vi "AlliGator Compute Natural Frequency.vi"(8 "Error In":errorcluster) -> (0 "Error Out":errorcluster, 3 "Natural Frequency":dbl[unit] caption="Laser Period" min=0.0 format="%#.3g")   [LabVIEW 2021, in "AlliGator Settings.lvlib"]
doc: "Computes the \"natural\" phasor frequency as a functions of various settings parameters."
uses:
  AlliGator Settings.lvlib
  AlliGator Settings List.ctl
  AlliGator Background Subtraction Parameters.ctl
  Graphs/XY Graph/XY Graph Plot Shift Parameters.ctl
  Graphs/XY Graph/XY Graph Plot Shift Method.ctl
  Variant/Variant to Data/Variant to U32.vi
  Variant/Variant to Data/Variant to Boolean.vi
  Variant/Variant to Data/Variant to Data.lvlib
  Graphs/XY Graph/XY Graph Add-Ons.lvlib
panel:
  # "see the AlliGator License on the block diagram (Ctrl+E or Window:Show Block Diagram)"
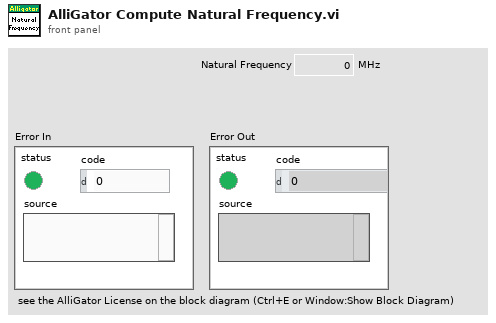
[diagram p1: front panel]
types:
  T1 = typedef "AlliGator Settings.lvlib/AlliGator Settings List.ctl" = enum16{"GUI:Visible Settings Tab", "GUI:Last Run Version", "Source Image:Use Image Histogram for Contrast", "Source Image:Low Count Pixels Rejection Options", "Source Image:High Count Pixels Rejection Options", "Source Image:Use Image Brightness", "Source Image:Blend Overlay with Image Background", "Source Image:Use Fixed ROI Diameter", "Source Image:ROI Diameter", "Source Image:ROI Center Color", "Source Image:Peak Threshold", "Source Image:Intensity Threshold", "Source Image:Image Binning Options", "Source Image:Image Smoothing Options", "Source Image:Image Histogram Active", "Source Image:Invert Binary Mask", "Source Image:Hot Pixel Removal", "Source Image:Overlay Analyzed ROI Center", "Source Image:Auto-Adjust Contrast", "Source Image:Histogram Lower Percentile", "Source Image:Histogram Upper Percentile", "Source Image:Save Source Image", "Source Image:Scale Bar Options", "Source Image:Image Resolution (Pixel Size)", "Source Image:Flatfield Correction", "Source Image:Show Dead Left Columns Correction", "Source Image:Dead Left Columns Correction", "Source Image:Image Pre-Processing Operations Order", "Source Image:Overlay ROI Median", "Source Image:Median Overlay Color", "Data Information:Gate Width", "Data Information:Nanotime Gate Separation", "Data Information:Macrotime Gate Separation", "Data Information:Gate Step", "Data Information:# Gates", "Data Information:Gate Image Exposure", "Data Information:Gate Image Integration", "Data Information:Gates to Skip", "Data Information:Gates to Keep", "Data Information:Define Gates to", "Data Information:Channel Name", "Data Information:Available Channel Names", "Data Information:Channel Arithmetic", "Data Information:Background File Subtraction", "Data Information:Background File", "Data Information:Background Scaling Factor", "Data Information:Background Pile-up Correction", "Data Information:Background Pixel Well Capacity", "Data Information:Laser Period", "Data Information:SYNC Period", "Data Information:Pile-up Correction", "Data Information:Pixel Well Capacity", "Data Information:Dataset Scaling Factor", "Fluorescence Decay_Decay Pre-Processing:Reverse Gates", "Fluorescence Decay_Decay Pre-Processing:Verbose Decay Pre-Processing", "Fluorescence Decay_Decay Pre-Processing:Use Decay Pre-Processing", "Fluorescence Decay_Decay Pre-Processing:Background Subtraction", "Fluorescence Decay_Decay Pre-Processing:Background Definition Range", "Fluorescence Decay_Decay Pre-Processing:Baseline Subtraction Method", "Fluorescence Decay_Decay Pre-Processing:Decay Pre-Processing Operations Order", "Fluorescence Decay_Decay Pre-Processing:Smoothing Parameter", "Fluorescence Decay_Decay Pre-Processing:Shift Decay", "Fluorescence Decay_Decay Pre-Processing:Decay Shift Parameters", "Fluorescence Decay_Decay Pre-Processing:Fold Decay", "Fluorescence Decay_Decay Pre-Processing:# Folds", "Fluorescence Decay_Decay Pre-Processing:1-Normalize Decay", "Fluorescence Decay_Decay Pre-Processing:[0-1]-Normalize Decay", "Fluorescence Decay_Decay Pre-Processing:Smoothen Decay", "Fluorescence Decay_Decay Pre-Processing:Extrapolate Decay", "Fluorescence Decay_Decay Pre-Processing:Use Periodicity", "Fluorescence Decay_Decay Pre-Processing:Use Cursors", "Fluorescence Decay_Decay Pre-Processing:Tail Fraction", "Fluorescence Decay_Decay Pre-Processing:Head Fraction", "Fluorescence Decay_Decay Pre-Processing:Additional Points", "Fluorescence Decay_Decay Pre-Processing:Straighten Decay", "Fluorescence Decay_Decay Pre-Processing:Constant Background", "Fluorescence Decay_Decay Pre-Processing:Pixel-Normalize Decay", "Fluorescence Decay_Advanced Analysis:Extract IRF instead of Decay", "Fluorescence Decay_Advanced Analysis:IRF Extraction Options", "Fluorescence Decay_Advanced Analysis:IRF Optimization Options", "Fluorescence Decay_Advanced Analysis:Square Pulse Options", "Fluorescence Decay_Advanced Analysis:IRF Order", "Fluorescence Decay_Advanced Analysis:IRF Time Constants", "Fluorescence Decay_Advanced Analysis:Wavelet Analysis Options", "Fluorescence Decay_Advanced Analysis:Average Lifetime Options", "Fluorescence Decay_Fit Options:Fit Options", "Fluorescence Decay_Fit Options:Use Legacy Fitting Approach", "Fluorescence Decay_Fit Options:Use Data Information Laser Period", "Fluorescence Decay_Fit Parameters:Displayed Fit Parameters", "Fluorescence Decay_Fit Parameters:Fit Parameter Constraints", "Fluorescence Decay_Fit Parameters:Export Tabulated Results", "Fluorescence Decay_Fit Parameters:MLE Baseline Offset Type", "Fluorescence Decay_Fit Parameters:MLE Baseline Offset", "Fluorescence Decay_Fit Parameters:Guess Parameter Names", "Fluorescence Decay_Fit Parameters:Guess Parameter Values", "Fluorescence Decay_Fit Parameters:Guess Parameters Options", "Fluorescence Decay_Styles:Show Last Decay Only", "Fluorescence Decay_Styles:Decay Graph Color Array", "Fluorescence Decay:Decay Graph Active", "Fluorescence Decay Statistics:Min Peak Value", "Fluorescence Decay Statistics:Reject Low Decay Peak Pixels", "Fluorescence Decay Statistics:Reject High Decay Peak Pixels", "Fluorescence Decay Statistics:Max Peak Value", "Time Traces:Use File Timestamp", "Time Traces:Time Step", "Time Traces:Use Intensity Correction File", "Time Traces:Intensity Correction File", "Phasor Plot:Phasor Plot Smoothing Options", "Phasor Plot:Phasor Plot Size", "Phasor Plot:Phasor Plot Graphics Options", "Phasor Plot:Cumulative Phasor Plot", "Phasor Plot:Use Phasor Brightness", "Phasor Plot:Blend Overlay with Phasor Background", "Phasor Plot:Save Phasor Plot", "Phasor Plot:Show References", "Phasor Plot:Phasor Ratio Decay Range", "Phasor Plot:Exponential Fading", "Phasor Plot:Phasor Ratio Reference Colors", "Phasor Plot:Reference Radius", "Phasor Plot:Show Color Map Vertices", "Phasor Plot:Phasor Plot Active", "Phasor Plot:Phasor Ratio Color Map Type", "Phasor Plot:Phasor Ratio Color Map", "Phasor Plot:Phasor Ratio Display Range", "Phasor Plot:Selected Image ROI(s)", "Phasor Plot:All Image ROIs", "Phasor Plot:Selected Phasor Plot ROI(s)", "Phasor Plot:All Phasor Plot ROIs", "Phasor Plot:Phasor Ratio Color-Coded Quantity", "Phasor Plot:Store Phasor Harmonics", "Phasor Plot:Draw Reference Segment", "Phasor Plot:User-Defined Quantity", "Phasor Graph:Phasor Frequency", "Phasor Graph:Phasor Ratio Type", "Phasor Graph:Pixel-level Phasor Computation", "Phasor Graph:Save Phasor Graph", "Phasor Graph:Phasor Graph Active", "Phasor Graph:Phasor SDV Options", "Phasor Calibration:Use Backup Calibration if needed", "Phasor Graph:Define Shortest Lifetime as", "Phasor Calibration:Backup Calibration Type", "Phasor Calibration:Calibration Type", "Phasor Calibration:Calibration Lifetime", "Phasor Calibration:Calibration Map Algorithm", "Single-Exponential Phasor Locus (SEPL):Gate Parameters", "Single-Exponential Phasor Locus (SEPL):User-defined Gate", "Single-Exponential Phasor Locus (SEPL):User-defined IRF", "Single-Exponential Phasor Locus (SEPL):Phasor Parameters", "Single-Exponential Phasor Locus (SEPL):Decay & IRF Parameters", "Single-Exponential Phasor Locus (SEPL):Display Parameters", "Lifetime Analysis:Decay Analysis Parameters", "Lifetime Analysis:Lifetime Map Active", "Plugins:Python Settings", "Miscellaneous:Verbose Mode", "Miscellaneous:Beep after Script", "Miscellaneous:Saved Image File Format", "Miscellaneous:Exported Gate Image Settings", "Miscellaneous:Include Loading in Timing", "Miscellaneous:Verbose Settings Mode", "Miscellaneous:Histogram Options", "Miscellaneous:Beep on Error", "Miscellaneous:# Logical Processors Used", "Miscellaneous:ROI Description Max Characters", "Miscellaneous:Verbose Error Mode", "Miscellaneous:Transparent Mask Color"}
  T2 = typedef "XY Graph Add-Ons.lvlib/XY Graph Plot Shift Parameters.ctl" = cluster{"Type":T3, "Shift":dbl[unit], "Threshold":dbl, "Rotate":bool}
  T3 = typedef "XY Graph Add-Ons.lvlib/XY Graph Plot Shift Method.ctl" = enum16{"Default", "CFD", "Threshold", "Cross-Correlation"}
  T4 = typedef "AlliGator Settings.lvlib/AlliGator Background Subtraction Parameters.ctl" = cluster{"Start":u32, "End":u32}
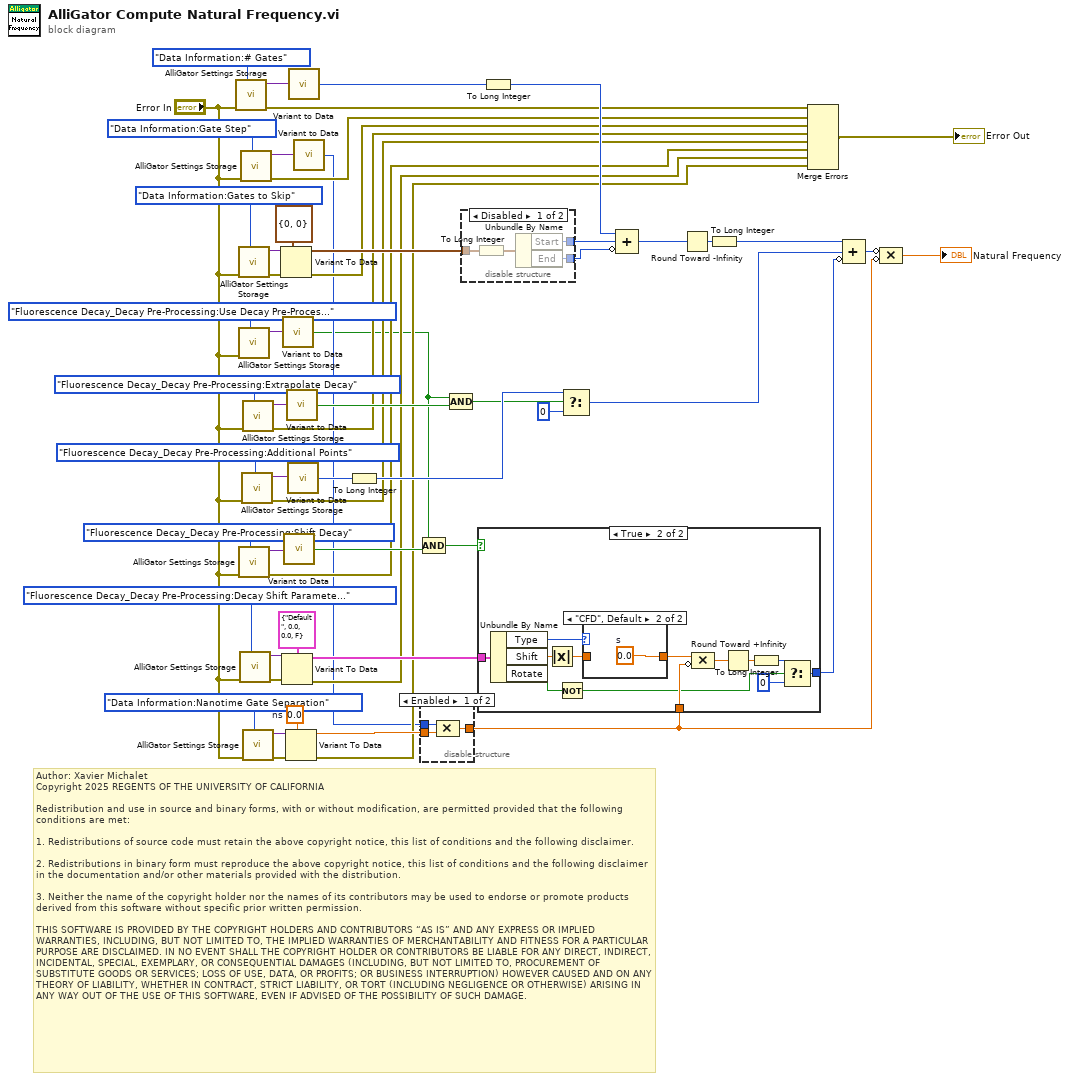
[diagram p0: block diagram]
diagram:
  w35 = dbl[unit] 0.0  # ns
  # "Author: Xavier Michalet\nCopyright 2025 REGENTS OF THE UNIVERSITY OF CALIFORNIA\n\nRedistribution and use in source and binary forms, with or without modification, are permitted provided that the following conditions are met:\n\n1. Redistributions of source code must retain the above copyright notice, this list of conditions and the following disclaimer.\n\n2. Redistributions in binary form must reproduce the above copyright notice, this list of conditions and the following disclaimer in the documentation and/or other materials provided with the distribution.\n\n3. Neither the name of the copyright holder nor the names of its contributors may be used to endorse or promote products derived from this software without specific prior written permission.\n\nTHIS SOFTWARE IS PROVIDED BY THE COPYRIGHT HOLDERS AND CONTRIBUTORS “AS IS” AND ANY EXPRESS OR IMPLIED WARRANTIES, INCLUDING, BUT NOT LIMITED TO, THE IMPLIED WARRANTIES OF MERCHANTABILITY AND FITNESS FOR A PARTICULAR PURPOSE ARE DISCLAIMED. IN NO EVENT SHALL THE COPYRIGHT HOLDER OR CONTRIBUTORS BE LIABLE FOR ANY DIRECT, INDIRECT, INCIDENTAL, SPECIAL, EXEMPLARY, OR CONSEQUENTIAL DAMAGES (INCLUDING, BUT NOT LIMITED TO, PROCUREMENT OF SUBSTITUTE GOODS OR SERVICES; LOSS OF USE, DATA, OR PROFITS; OR BUSINESS INTERRUPTION) HOWEVER CAUSED AND ON ANY THEORY OF LIABILITY, WHETHER IN CONTRACT, STRICT LIABILITY, OR TORT (INCLUDING NEGLIGENCE OR OTHERWISE) ARISING IN ANY WAY OUT OF THE USE OF THIS SOFTWARE, EVEN IF ADVISED OF THE POSSIBILITY OF SUCH DAMAGE."
  n1 = call "AlliGator Settings Storage.vi"("AlliGator Settings List"=AlliGator_Settings_List."Data Information:# Gates", "Error In"="Error In") -> ("Error Out"=w18:errorcluster, "Variant Data out"=w52:variant)  [unwired: 8 in]
  n2 = call "AlliGator Settings Storage.vi"("AlliGator Settings List"=AlliGator_Settings_List."Data Information:Gates to Skip", "Error In"="Error In") -> ("Error Out"=w50:errorcluster, "Variant Data out"=w51:variant)  [unwired: 8 in]
  n3 = call "AlliGator Settings Storage.vi"("AlliGator Settings List"=AlliGator_Settings_List."Fluorescence Decay_Decay Pre-Processing:Use Decay Pre-Processing", "Error In"="Error In") -> ("Variant Data out"=w6:variant)  [unwired: 8 in, 1 out]
  n4 = call "AlliGator Settings Storage.vi"("AlliGator Settings List"=AlliGator_Settings_List."Fluorescence Decay_Decay Pre-Processing:Shift Decay", "Error In"="Error In") -> ("Error Out"=w13:errorcluster, "Variant Data out"=w48:variant)  [unwired: 8 in]
  n5 = call "AlliGator Settings Storage.vi"("AlliGator Settings List"=AlliGator_Settings_List."Fluorescence Decay_Decay Pre-Processing:Decay Shift Parameters", "Error In"="Error In") -> ("Error Out"=w46:errorcluster, "Variant Data out"=w47:variant)  [unwired: 8 in]
  n6 = call "AlliGator Settings Storage.vi"("AlliGator Settings List"=AlliGator_Settings_List."Data Information:Gate Step", "Error In"="Error In") -> ("Error Out"=w17:errorcluster, "Variant Data out"=w40:variant)  [unwired: 8 in]
  n7 = call "AlliGator Settings Storage.vi"("AlliGator Settings List"=AlliGator_Settings_List."Fluorescence Decay_Decay Pre-Processing:Additional Points", "Error In"="Error In") -> ("Error Out"=w14:errorcluster, "Variant Data out"=w43:variant)  [unwired: 8 in]
  n8 = call "AlliGator Settings Storage.vi"("AlliGator Settings List"=AlliGator_Settings_List."Fluorescence Decay_Decay Pre-Processing:Extrapolate Decay", "Error In"="Error In") -> ("Error Out"=w15:errorcluster, "Variant Data out"=w44:variant)  [unwired: 8 in]
  n9 = call "AlliGator Settings Storage.vi"("AlliGator Settings List"=AlliGator_Settings_List."Data Information:Nanotime Gate Separation", "Error In"="Error In") -> ("Error Out"=w37:errorcluster, "Variant Data out"=w36:variant)  [unwired: 8 in]
  n10 = Variant To Data(error in=w50, type=T4 {"Start"=0, "End"=0} ("Gates to Skip"), Variant=w51) -> (data=w42:T4, error out=w16:errorcluster)
  n11 = Variant To Data(error in=w46, type=T2 {"Type"=enum."Default", "Shift"=0.0, "Threshold"=0.0, "Rotate"=FALSE} ("IRF Analysis Parameters"), Variant=w47) -> (data=w41:T2, error out=w12:errorcluster)
  n12 = call-poly "Variant to Data.vi"("Variant"=w6) -> ("Value"=w1:bool)  [unwired: 8 in]
  n13 = call-poly "Variant to Data.vi"("Variant"=w48) -> ("Value"=w30:bool)  [unwired: 8 in]
  n14 = Variant To Data(error in=w37, type=w35, Variant=w36) -> (data=w20:dbl[unit], error out=w11:errorcluster)
  n15 = call-poly "Variant to Data.vi"("Variant"=w44) -> ("Value"=w29:bool)  [unwired: 8 in]
  n16 = call-poly "Variant to Data.vi"("Variant"=w43) -> ("Value"=w28:u32)  [unwired: 8 in]
  n17 = call-poly "Variant to Data.vi"("Variant"=w52) -> ("Value"=w34:u32)  [unwired: 8 in]
  n18 = call-poly "Variant to Data.vi"("Variant"=w40) -> ("Value"=w7:u32)  [unwired: 8 in]
  n19 = To Long Integer(number=w28) -> (32bit integer=w27:i32)
  n20 = disable-structure shown="Enabled" {
    disable-tunnel: w20 -> [w61 w62]
    disable-tunnel: [w60 w62] -> w9
    disable-tunnel: w7 -> [w59 _]
    frame Enabled {
      n21 = Compound Arithmetic op=MULTIPLY(w59, w61) -> (w60:dbl[unit])
    }
    frame Disabled {
    }
  }
  n22 = Compound Arithmetic op=AND(w1, w30) -> (w3:bool)
  n23 = Compound Arithmetic op=AND(w1, w29) -> (w2:bool)
  n24 = disable-structure shown="Disabled" {
    disable-tunnel: w42 -> [w66 _]
    disable-tunnel: [w65 _] -> w33
    disable-tunnel: [w63 _] -> w31
    frame Disabled {
      n25 = To Long Integer(number=w66) -> (32bit integer=w64:cluster{"Start":i32, "End":i32})
      n26 = Unbundle By Name(w64) -> ("Start"=w65:i32, "End"=w63:i32)
    }
    frame Enabled {
    }
  }
  n27 = case shown="True" w3 {
    tunnel: w41 -> [_ w79]
    tunnel: w9 -> [_ w73]
    tunnel: [_ w68] -> w22
    frame False {
    }
    frame True {
      n28 = Unbundle By Name(w79) -> ("Type"=w78:T3, "Shift"=w77:dbl[unit], "Rotate"=w75:bool)
      n29 = Absolute Value(x=w77) -> (abs(x)=w76:dbl[unit])
      n30 = Not(x=w75) -> (.not. x?=w67:bool)
      n31 = case shown="\"CFD\", Default" w78 {
        tunnel: w76 -> [w80 _]
        tunnel: [w80 w81] -> w74
        frame "Default" {
        }
        frame "CFD", Default {
          w81 = dbl[unit] 0.0  # s
        }
      }
      n32 = Compound Arithmetic op=MULTIPLY(w74, invert w73) -> (w72:dbl)
      n33 = Round Toward +Infinity(x=w72) -> (ceil(x): smallest int >= x=w70:dbl)
      n34 = To Long Integer(number=w70) -> (32bit integer=w69:i32)
      n35 = Select(t=w69, s=w67, f=0) -> (s? t:f=w68:i32)
    }
  }
  n36 = To Long Integer(number=w34) -> (32bit integer=w32:i32)
  n37 = Select(t=w27, s=w2, f=0) -> (s? t:f=w23:i32)
  n38 = Compound Arithmetic op=ADD(w32, w33, invert w31) -> (w8:i32)
  n39 = Round Toward -Infinity(1:w8) -> (0:w25:i32)
  n40 = To Long Integer(number=w25) -> (32bit integer=w24:i32)
  n41 = Merge Errors(w18, w17, w16, w15, w14, w13, w12, w11) -> (→"Error Out":errorcluster)
  n42 = Compound Arithmetic op=ADD(w24, w23, invert w22) -> (w21:i32)
  n43 = Compound Arithmetic op=MULTIPLY(invert w21, invert w9) -> (→"Natural Frequency":dbl[unit])
